vi "Add Peak and Valley Detection Settings Section.vi"(8 "error in (no error)":errorcluster, 10 "Stages":string[](array[string])=["Boost", "Battery", "Off"], 11 "Global Settings Item Ref in":T1=18446744073709551615 format="%.0x") -> (0 "error out":errorcluster, 3 "Global Settings Item Ref out":T1=18446744073709551615 format="%.0x")   [LabVIEW 2015, in "Fuel Injection Addon System Explorer.lvlib"]
uses:
  Fuel Injection Addon System Explorer.lvlib
  <vilib>/NI Veristand/Custom Device API/Custom Device Item Ref.ctl
  Shared/Types/Analysis.Channels.Select.ctl
  <vilib>/NI Veristand/Custom Device API/Custom Device Channel.ctl
  <vilib>/NI Veristand/Custom Device API/Custom Device Channel Type.ctl
  Shared/Types/Stage.PullIn.Types.ctl
  Shared/Types/Stage.Transition.Types.ctl
  Shared/Constants.vi
  <vilib>/NI Veristand/Custom Device Tools/Custom Device Utility Library/NI VeriStand - Search for Item by GUID.vi
  <vilib>/NI VeriStand/Custom Device API/Custom Device API.lvlib
  Shared/Fuel Injection Addon Shared.lvlib
  <vilib>/NI Veristand/Custom Device Tools/Custom Device Utility Library/Custom Device Utility Library.lvlib
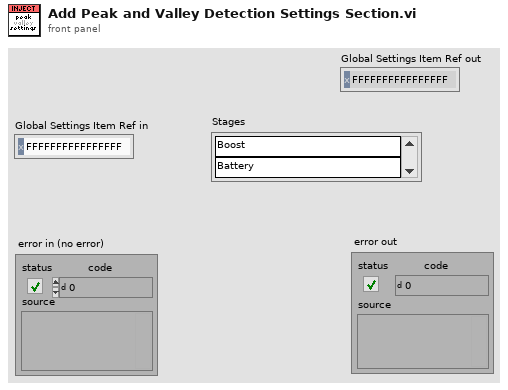
[diagram p1: front panel]
types:
  T1 = typedef "Custom Device API.lvlib/Custom Device Item Ref.ctl" = u64
  T2 = typedef "Fuel Injection Addon Shared.lvlib/Stage.Transition.Types.ctl" = enum8{"Stage Transition Dwell Time", "Stage Transition Voltage Level", "Stage Transition Current Drop"}
  T3 = typedef "Fuel Injection Addon Shared.lvlib/Stage.PullIn.Types.ctl" = enum8{"Pull In Transition Dwells", "Pull In Transition Current Drop"}
  T4 = typedef "Fuel Injection Addon Shared.lvlib/Analysis.Channels.Select.ctl" = cluster{"Pull In Time":bool, "Pull In Max Current":bool, "Hold In Time":bool, "Hold In Max Current":bool, "Hold In Min Current":bool, "Hold In Avg Current":bool, "Hold In Avg Max Current":bool, "Hold In Avg Min Current":bool, "Hold In Max Voltage":bool, "Hold In Min Voltage":bool, "Hold In Avg Voltage":bool, "Hold In Avg Max Voltage":bool, "Hold In Avg Min Voltage":bool, "Off Time":bool, "Off Stage Max Current":bool, "Off Stage Min Current":bool, "Off Stage Avg Current":bool, "Total Voltage Pulses":bool}
  T5 = typedef "Custom Device API.lvlib/Custom Device Channel.ctl" = cluster{"Type":T6, "Units":string, "Default Value":dbl, "Faultable":bool, "Scalable":bool}
  T6 = typedef "Custom Device API.lvlib/Custom Device Channel Type.ctl" = enum16{"Input", "Output"}
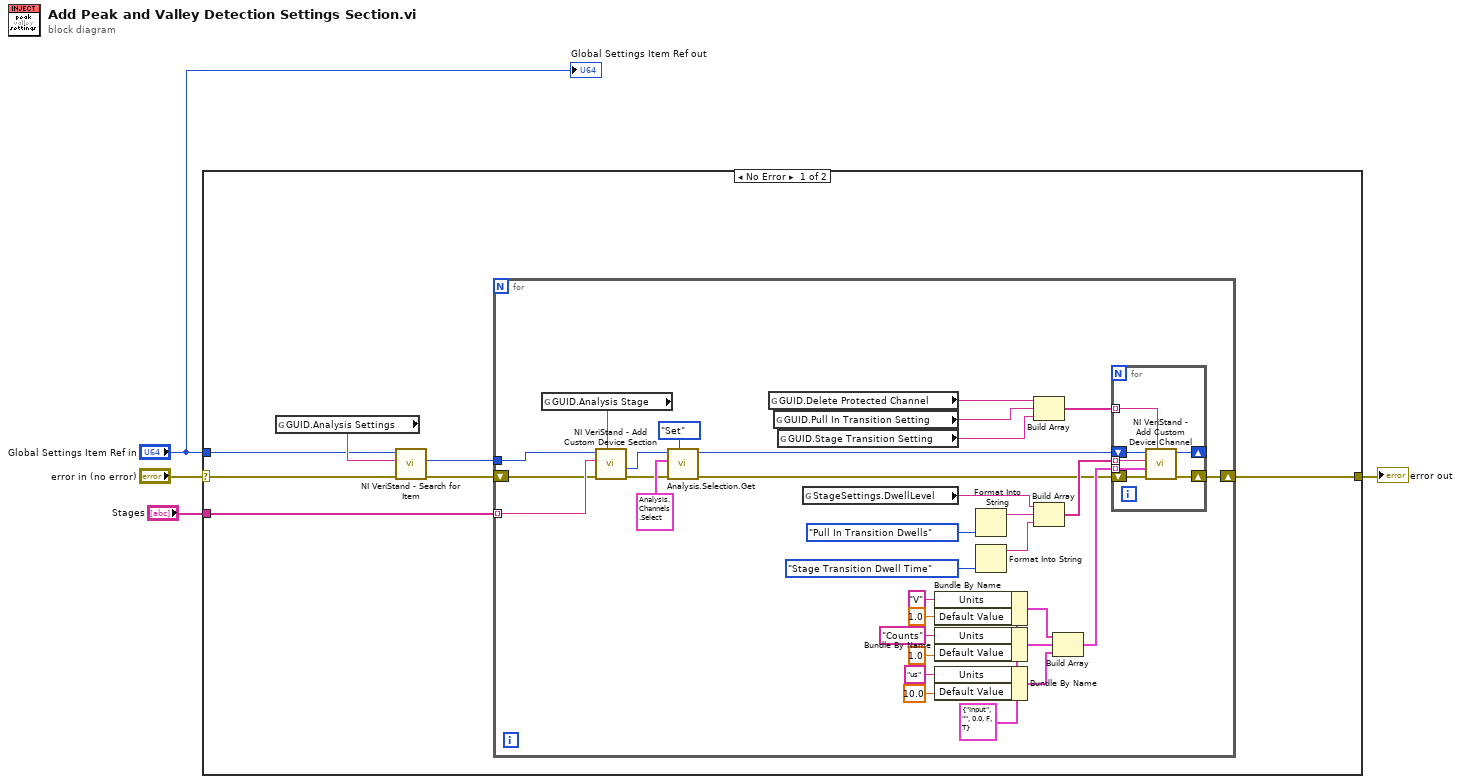
[diagram p0: block diagram]
diagram:
  n1 = case shown="No Error" "error in (no error)" {
    selector: "error in (no error)" -> [w8 w51]
    tunnel: [w11 w51] -> w3
    tunnel: "Global Settings Item Ref in" -> [w7 _]
    tunnel: "Stages" -> [w10 _]
    frame No Error {
      n2 = global read "Constants.vi" "GUID.Analysis Settings"() -> (w9:string)
      n3 = call-poly <vilib>:"NI VeriStand - Search for Item.vi"("error in"=w8, "Item GUID"=w9, "Section Ref in"=w7) -> ("error out"=w6:errorcluster, "Item Ref"=w5:T1)  [unwired: 5 in, 2 out]
      n4 = for {
        shift-right: [w31] -> w11
        shift-left: w6 -> [w41]
        tunnel: w10 -> [w42] mode=indexing
        tunnel: w5 -> [w40]
        w24 = T5 {"Type"=enum."Input", "Units"="", "Default Value"=0.0, "Faultable"=FALSE, "Scalable"=TRUE} ("Channel")
        n5 = global read "Constants.vi" "GUID.Analysis Stage"() -> (w43:string)
        n6 = call <vilib>:"NI VeriStand - Add Custom Device Section.vi"("GUID (Default Section)"=w43, "error in (no error)"=w41, "Section Name"=w42, "Parent Ref in"=w40) -> ("error out"=w37:errorcluster, "Section Ptr"=w38:T1)  [unwired: 4 in, 2 out]
        n7 = call "Analysis.Selection.Get.vi"("Action"=enum8{"Get", "Set"}."Set", "error in (no error)"=w37, "Selections"=T4 {"Pull In Time"=TRUE, "Pull In Max Current"=TRUE, "Hold In Time"=TRUE, "Hold In Max Current"=TRUE, "Hold In Min Current"=TRUE, "Hold In Avg Current"=TRUE, "Hold In Avg Max Current"=TRUE, "Hold In Avg Min Current"=TRUE, "Hold In Max Voltage"=TRUE, "Hold In Min Voltage"=TRUE, "Hold In Avg Voltage"=TRUE, "Hold In Avg Max Voltage"=TRUE, "Hold In Avg Min Voltage"=TRUE, "Off Time"=TRUE, "Off Stage Max Current"=TRUE, "Off Stage Min Current"=TRUE, "Off Stage Avg Current"=TRUE, "Total Voltage Pulses"=TRUE} ("Analysis Options"), "Item Ref in"=w38) -> ("error out"=w18:errorcluster, "Item Ref out"=w19:T1)  [unwired: 5 in, 1 out]
        n8 = global read "Constants.vi" "GUID.Delete Protected Channel"() -> (w15:string)
        n9 = global read "Constants.vi" "GUID.Pull In Transition Setting"() -> (w14:string)
        n10 = global read "Constants.vi" "GUID.Stage Transition Setting"() -> (w13:string)
        n11 = global read "Constants.vi" "StageSettings.DwellLevel"() -> (w26:string)
        n12 = Bundle By Name(cluster=w24, "Units"="V", "Default Value"=1.0) -> (w25:T5)
        n13 = Bundle By Name(cluster=w24, "Units"="Counts", "Default Value"=1.0) -> (w32:T5)
        n14 = Bundle By Name(cluster=w24, "Units"="us", "Default Value"=10.0) -> (w33:T5)
        n15 = Format Into String(Stage.PullIn.Types."Pull In Transition Dwells" ("input 1")) -> (resulting string=w20:string)  [unwired: 3 in, 1 out]
        n16 = Format Into String(Stage.Transition.Types."Stage Transition Dwell Time" ("input 1")) -> (resulting string=w21:string)  [unwired: 3 in, 1 out]
        n17 = Build Array(w15, w14, w13) -> (w12:string[])
        n18 = Build Array(w26, w20, w21) -> (w35:string[])
        n19 = Build Array(w25, w32, w33) -> (w34:T5[])
        n20 = for {
          shift-right: [w49] -> w31
          shift-left: w18 -> [w50]
          tunnel: w34 -> [w47] mode=indexing
          tunnel: w12 -> [w46] mode=indexing
          tunnel: w35 -> [w45] mode=indexing
          shift-right: [w44] -> _
          shift-left: w19 -> [w48]
          n21 = call <vilib>:"NI VeriStand - Add Custom Device Channel.vi"("GUID (Default Channel)"=w46, "error in (no error)"=w50, "Channel"=w47, "Channel Name"=w45, "Parent Ref in"=w48) -> ("error out"=w49:errorcluster, "Parent Ref out"=w44:T1)  [unwired: 3 in, 2 out]
        }
      }
    }
    frame Error {
    }
  }
  "error out" <- w3
  "Global Settings Item Ref out" <- "Global Settings Item Ref in"
